vi "Set Acquisition Mode.vi"(8 "error in (no error)":errorcluster, 11 "CCDCamera in":refnum<class "CCDCamera.lvclass">) -> (0 "error out":errorcluster, 3 "CCDCamera out":refnum<class "CCDCamera.lvclass">)   [LabVIEW 2018, in "CCDCamera.lvclass"]
doc: "Set the image acquisition mode (single scan or kinetic)"
uses:
  CCDCamera.lvclass
  C:/Users/observer/Desktop/SPARC4_ACS/SPARC4_ACS/Simulated_CCD_Camera/Simulated_CCD_Camera.lvclass
  Simulated_CCD_Camera/Simulated_CCD_Camera.lvclass
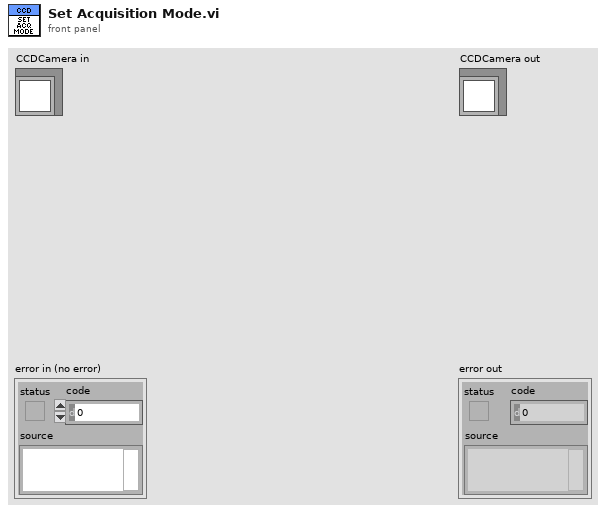
[diagram p1: front panel]
types:
  T1 = cluster{"PREAMP":u16, "READOUT_RATE":u16, "EM_GAIN":u16, "VERTICAL_SHIFT_SPEED":u16, "READ_MODE":u16, "FRAME_TRANSFER":bool, "VERTICAL_CLOCK_VOLTAGE":u16, "ACQUISITION_MODE":u16, "AD_CHANNEL":u16, "EM_MODE":u16, "SHUTTER_TTL":u16, "SHUTTER_OPENING_TIME":u16, "SHUTTER_CLOSING_TIME":u16, "SHUTTER_MODE":u16, "TRIGGER_MODE":u16, "VBIN":u16, "INITIAL_LINE":u16, "INITIAL_COLUMN":u16, "FINAL_LINE":u16, "FINAL_COLUMN":u16, "HBIN":u16}
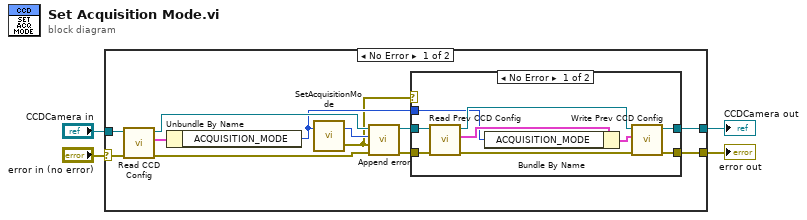
[diagram p0: block diagram]
diagram:
  n1 = case shown="No Error" "error in (no error)" {
    selector: "error in (no error)" -> [w16 w29]
    tunnel: [w6 w29] -> w4
    tunnel: [w7 w28] -> w3
    tunnel: "CCDCamera in" -> [w14 w28]
    frame No Error {
      n2 = call "Read CCD Config.vi"("error in (no error)"=w16, "CCDCamera in"=w14) -> ("error out"=w12:errorcluster, "CCD Config"=w15:T1, "CCDCamera out"=w13:refnum<class "CCDCamera.lvclass">)  [unwired: 7 in]
      n3 = Unbundle By Name(w15) -> ("ACQUISITION_MODE"=w8:u16)
      n4 = call <userlib>:"SetAcquisitionMode.vi"("mode"=w8) -> ("error out"=w5:errorcluster, "DLL error code"=w11:u32)  [unwired: 1 in]
      n5 = call "Append error.vi"("error in (no error)"=w12, "error"=w5, "code"=w11, "Simulated_CCD_Camera in"=w13) -> ("error out"=w9:errorcluster, "Simulated_CCD_Camera out"=w10:refnum<class "CCDCamera.lvclass">)  [unwired: 6 in]
      n6 = case shown="No Error" w5 {
        tunnel: [w24 w27] -> w7
        tunnel: [w22 w26] -> w6
        tunnel: w10 -> [w19 w27]
        tunnel: w9 -> [w17 w26]
        tunnel: w8 -> [w18 _]
        frame No Error {
          n7 = call-dynamic "Read Prev CCD Config.vi"("error in (no error)"=w17, "Simulated_CCD_Camera in"=w19) -> ("error out"=w23:errorcluster, "Prev CCD Config"=w21:T1, "Simulated_CCD_Camera out"=w25:refnum<class "CCDCamera.lvclass">)  [unwired: 7 in]
          n8 = Bundle By Name(cluster=w21, "ACQUISITION_MODE"=w18) -> (w20:T1)
          n9 = call-dynamic "Write Prev CCD Config.vi"("error in (no error)"=w23, "Prev CCD Config"=w20, "Simulated_CCD_Camera in"=w25) -> ("error out"=w22:errorcluster, "Simulated_CCD_Camera out"=w24:refnum<class "CCDCamera.lvclass">)  [unwired: 7 in]
        }
        frame Error {
        }
      }
    }
    frame Error {
    }
  }
  "error out" <- w4
  "CCDCamera out" <- w3
